vi "ROI grp-Set POI grouping window state.vi"(8 "error in (no error)":errorcluster, 11 "Front Panel Window:State":T1(ring)) -> (0 "error out":errorcluster)   [LabVIEW 2020]
uses:
  Globals/gl_ROI grp window globals.vi
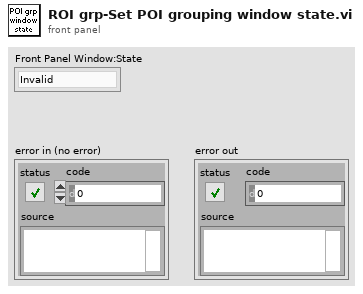
[diagram p1: front panel]
types:
  T1 = enum32{"Invalid", "Standard", "Closed", "Hidden", "Minimized", "Maximized"}
  T2 = typedef "ROI grp-window ctrl refs.ctl" = cluster{"This VI":refnum<vi>, "Pane":refnum<vi>, "Table":refnum<vi>}
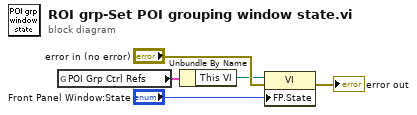
[diagram p0: block diagram]
diagram:
  n1 = global read "gl_ROI grp window globals.vi" "POI Grp Ctrl Refs"() -> (w1:T2)
  n2 = Unbundle By Name(w1) -> ("This VI"=w2:refnum<vi>)
  n3 = property on="Property Node" class="VI"(reference=w2, error in="error in (no error)", "FP.State"="Front Panel Window:State") -> (error out=→"error out":errorcluster)  [unwired: 1 out]
